vi "reward_behavior_timeout_phase1_2.vi"() -> ()   [LabVIEW 2019]
doc: "The myRIO Project template acquires acceleration data from the onboard accelerometer and displays the changes of acceleration values in a waveform chart."
uses:
  <vilib>/Analysis/Matrix/Datatypes/RealMatrix.ctl
  <vilib>/myRIO/Common/Instrument Driver Framework/myRIO v1.0/Encoder/typedefs/Encoder Signal Mode.ctl
  <vilib>/myRIO/Instrument Drivers/Onboard IO/Encoder/typedefs/Encoder Reference.ctl
  <vilib>/myRIO/Common/Instrument Driver Framework/Utilities/typedefs/myRIO Generic Hardware Reference.ctl
  <vilib>/myRIO/Common/Instrument Driver Framework/Utilities/typedefs/Hardware Version Enum.ctl
  <vilib>/myRIO/Common/Instrument Driver Framework/Utilities/typedefs/myRIO v1.0 Reference.ctl
  <vilib>/myRIO/Common/Instrument Driver Framework/Utilities/typedefs/Generic FPGA Reference.ctl
  <vilib>/myRIO/Common/Instrument Driver Framework/myRIO v1.0/Encoder/typedefs/Encoder Channels Enum.ctl
  <vilib>/myRIO/Common/Instrument Driver Framework/myRIO v1.0/Encoder/typedefs/Encoder Configuration v1.0.ctl
  <vilib>/userdefined/High Color/nirio_resource_hc.ctl
  <vilib>/myRIO/Instrument Drivers/Onboard IO/DIO/typedefs/DIO Reference.ctl
  <vilib>/myRIO/Common/Instrument Driver Framework/myRIO v1.0/DIO/typedefs/DIO Channels List.ctl
  <vilib>/myRIO/Common/Instrument Driver Framework/myRIO v1.0/DIO/typedefs/DIO Channels Enum.ctl
  <vilib>/myRIO/Common/Instrument Driver Framework/Utilities/vis/Is FPGA Ref Available.vi
  <vilib>/myRIO/Common/Instrument Driver Framework/myRIO v1.0/Encoder/vis/myRIO v1.1 Open Encoder.vi
  <vilib>/myRIO/Instrument Drivers/Onboard IO/Encoder/vis/Read.vi
  <vilib>/myRIO/Common/Instrument Driver Framework/myRIO v1.0/DIO/vis/myRIO v1.1 Open DIO.vi
  <vilib>/myRIO/Instrument Drivers/Onboard IO/DIO/vis/Write.vi
  <vilib>/myRIO/Instrument Drivers/Onboard IO/DIO/vis/Read.vi
  <vilib>/myRIO/Common/Instrument Driver Framework/Utilities/vis/Validate Channels.vi
  <vilib>/myRIO/Common/Instrument Driver Framework/myRIO v1.0/Encoder/vis/myRIO v1.0 Reserve Encoder.vi
  <vilib>/myRIO/Common/Instrument Driver Framework/myRIO v1.0/DIO/vis/myRIO v1.0 Reserve DIO.vi
  <vilib>/myRIO/Common/Instrument Driver Framework/myRIO v1.0/Encoder/vis/myRIO v1.0 Build MUX Configuration Encoder.vi
  <vilib>/myRIO/Common/Instrument Driver Framework/myRIO v1.0/Resource Manager/vis/myRIO v1.0 Reserve Channel List.vi
  <vilib>/myRIO/Common/Instrument Driver Framework/myRIO v1.0/DIO/vis/myRIO v1.0 Build MUX Configuration DIO.vi
  <vilib>/myRIO/Common/Instrument Driver Framework/myRIO v1.0/Resource Manager/vis/myRIO v1.0 Create Configuration List.vi
  <vilib>/myRIO/Common/Instrument Driver Framework/myRIO v1.0/Resource Manager/vis/myRIO v1.0 Reserve Channel.vi
  <vilib>/myRIO/Common/Instrument Driver Framework/myRIO v1.0/Resource Manager/vis/myRIO v1.0 Unreserve Channel.vi
  <vilib>/myRIO/Common/Instrument Driver Framework/myRIO v1.0/Resource Manager/vis/myRIO v1.0 Build Mutex Name.vi
  <vilib>/Utility/VariantDataType/GetNumericInfo.vi
  <vilib>/Utility/error.llb/Error Cluster From Error Code.vi
  <vilib>/myRIO/Common/Instrument Driver Framework/myRIO v1.0/myRIO v1.1 Open.vi
  <vilib>/myRIO/Common/Instrument Driver Framework/Utilities/vis/IO Manager.vi
  <vilib>/myRIO/Common/Instrument Driver Framework/Utilities/vis/Configuration Manager.vi
  <vilib>/myRIO/Common/Instrument Driver Framework/myRIO v1.0/Resource Manager/vis/myRIO v1.0 Configure IO.vi
  <vilib>/myRIO/Common/Instrument Driver Framework/myRIO v1.0/myRIO v1.0 Close.vi
  <vilib>/myRIO/Common/Instrument Driver Framework/myRIO v1.0/Encoder/vis/myRIO v1.0 Configure Encoder.vi
  <vilib>/myRIO/Common/Instrument Driver Framework/myRIO v1.0/Encoder/vis/myRIO v1.0 Read Encoder.vi
  <vilib>/myRIO/Common/Instrument Driver Framework/myRIO v1.0/DIO/vis/myRIO v1.0 Read DIO.vi
  <vilib>/myRIO/Common/Instrument Driver Framework/myRIO v1.0/DIO/vis/myRIO v1.0 Write DIO.vi
  <vilib>/myRIO/Express VI/Onboard IO/Encoder/Encoder Express VI.xnode
  <vilib>/myRIO/Instrument Drivers/Onboard IO/Encoder/vis/myRIO Encoder Open.xnode
  <vilib>/myRIO/Express VI/Onboard IO/DI/DI Express VI.xnode
  <vilib>/myRIO/Instrument Drivers/Onboard IO/DIO/vis/myRIO DIO Open.xnode
  <vilib>/myRIO/Express VI/Onboard IO/DO/DO Express VI.xnode
  <vilib>/myRIO/Instrument Drivers/Onboard IO/Encoder/Encoder.lvlib
  <vilib>/myRIO/Instrument Drivers/Onboard IO/DIO/DIO.lvlib
  <vilib>/Analysis/Matrix/NI_Matrix.lvlib
panel:
  out "Timings":dbl[](array[numeric])
  out "ISI":dbl
  out "ISI start time":dbl
  out "Time_out":bool=TRUE
  out "Time since lick":dbl
  out "Time of last lick":dbl
  out "Rewarded trials":dbl[](array[numeric])
  out "Rewards":u16
  out "Active Trial":bool
  out "Array temp2":T1
  out "Stimuli Loaded":bool
  out "Stim_ID":dbl[](array[numeric])
  out "Reward_mat":dbl[](array[numeric])
  out "Reward":bool=TRUE
  out "Frame clock":i32
  out "Licks":u32
  out "Lick":bool
  out "Time":dbl
  out "Stop":bool
  in  "Frames to collect":u32
  out "Overflow?":bool
  out "Counter Value":i32
  out "Velocity":dbl
  out "Velocity Plot":dbl[](graph)
  out "Velocity array":dbl[](array[numeric])
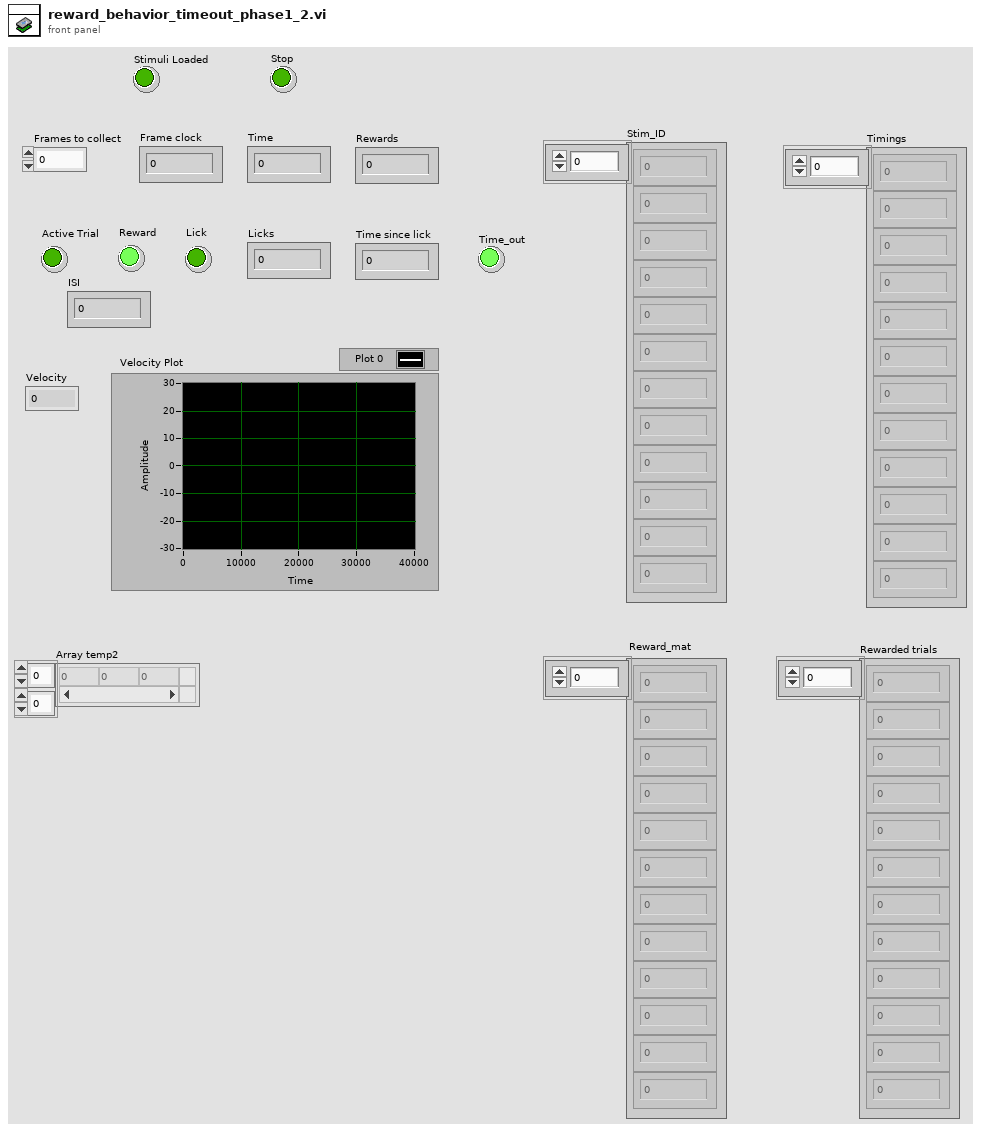
[diagram p1: front panel]
types:
  T1 = typedef "NI_Matrix.lvlib/RealMatrix.ctl" = dbl[][]
  T2 = typedef "Encoder.lvlib/Encoder Reference.ctl" = cluster{"myRIO Reference":T3, "Encoder Channels Enum":T7}
  T3 = typedef "myRIO Generic Hardware Reference.ctl" = cluster{"myRIO Model":T4, "myRIO Hardware Reference":T5}
  T4 = typedef "Hardware Version Enum.ctl" = enum16{"Unknown", "myRIO-1900", "myRIO-1950", "roboRIO", "NI ELVIS RIO CM", "ELVIS III"}
  T5 = typedef "myRIO v1.0 Reference.ctl" = cluster{"Generic FPGA Reference":T6, "Allow multiple opens":bool}
  T6 = typedef "Generic FPGA Reference.ctl" = refnum<k20>
  T7 = typedef "Encoder Channels Enum.ctl" = enum16{"Not Connected", "C/ENC0", "C/ENC1", "A/ENC", "A/ENC0", "A/ENC1", "A/ENC2", "A/ENC3", "A/ENC4", "A/ENC5", "A/ENC6", "A/ENC7", "A/ENC8", "A/ENC9", "B/ENC", "B/ENC0", "B/ENC1", "B/ENC2", "B/ENC3", "B/ENC4", "B/ENC5", "B/ENC6", "B/ENC7", "B/ENC8", "B/ENC9", "DIO/ENC0", "DIO/ENC1", "DIO/ENC2", "DIO/ENC3", "DIO/ENC4"}
  T8 = typedef "Encoder Signal Mode.ctl" = enum16{"Quadrature phase signal", "Step and direction signal"}
  T9 = typedef "nirio_resource_hc.ctl" = tag
  T10 = typedef "DIO.lvlib/DIO Reference.ctl" = cluster{"myRIO Reference":T3, "DIO Channels List":T11}
  T11 = typedef "DIO Channels List.ctl" = T12[]
  T12 = typedef "DIO Channels Enum.ctl" = enum16{"Not Connected", "C/DIO0", "C/DIO1", "C/DIO2", "C/DIO3", "C/DIO4", "C/DIO5", "C/DIO6", "C/DIO7", "A/DIO0", "A/DIO1", "A/DIO2", "A/DIO3", "A/DIO4", "A/DIO5", "A/DIO6", "A/DIO7", "A/DIO8", "A/DIO9", "A/DIO10", "A/DIO11", "A/DIO12", "A/DIO13", "A/DIO14", "A/DIO15", "A/DIO16", "A/DIO17", "A/DIO18", "A/DIO19", "B/DIO0", "B/DIO1", "B/DIO2", "B/DIO3", "B/DIO4", "B/DIO5", "B/DIO6", "B/DIO7", "B/DIO8", "B/DIO9", "B/DIO10", "B/DIO11", "B/DIO12", "B/DIO13", "B/DIO14", "B/DIO15", "B/DIO16", "B/DIO17", "B/DIO18", "B/DIO19", "LED0", "LED1", "LED2", "LED3", "Button0", "DIO/DIO0", "DIO/DIO1", "DIO/DIO2", "DIO/DIO3", "DIO/DIO4", "DIO/DIO5", "DIO/DIO6", "DIO/DIO7", "DIO/DIO8", "DIO/DIO9", "SPI/CS0", "SPI/CS1", "SPI/CS2", "SPI/CS3", "LED RADIO (Green)", "LED RADIO (Red)", "LED COMM (Green)", "LED COMM (Red)", "LED MODE (Green)", "LED MODE (Red)"}
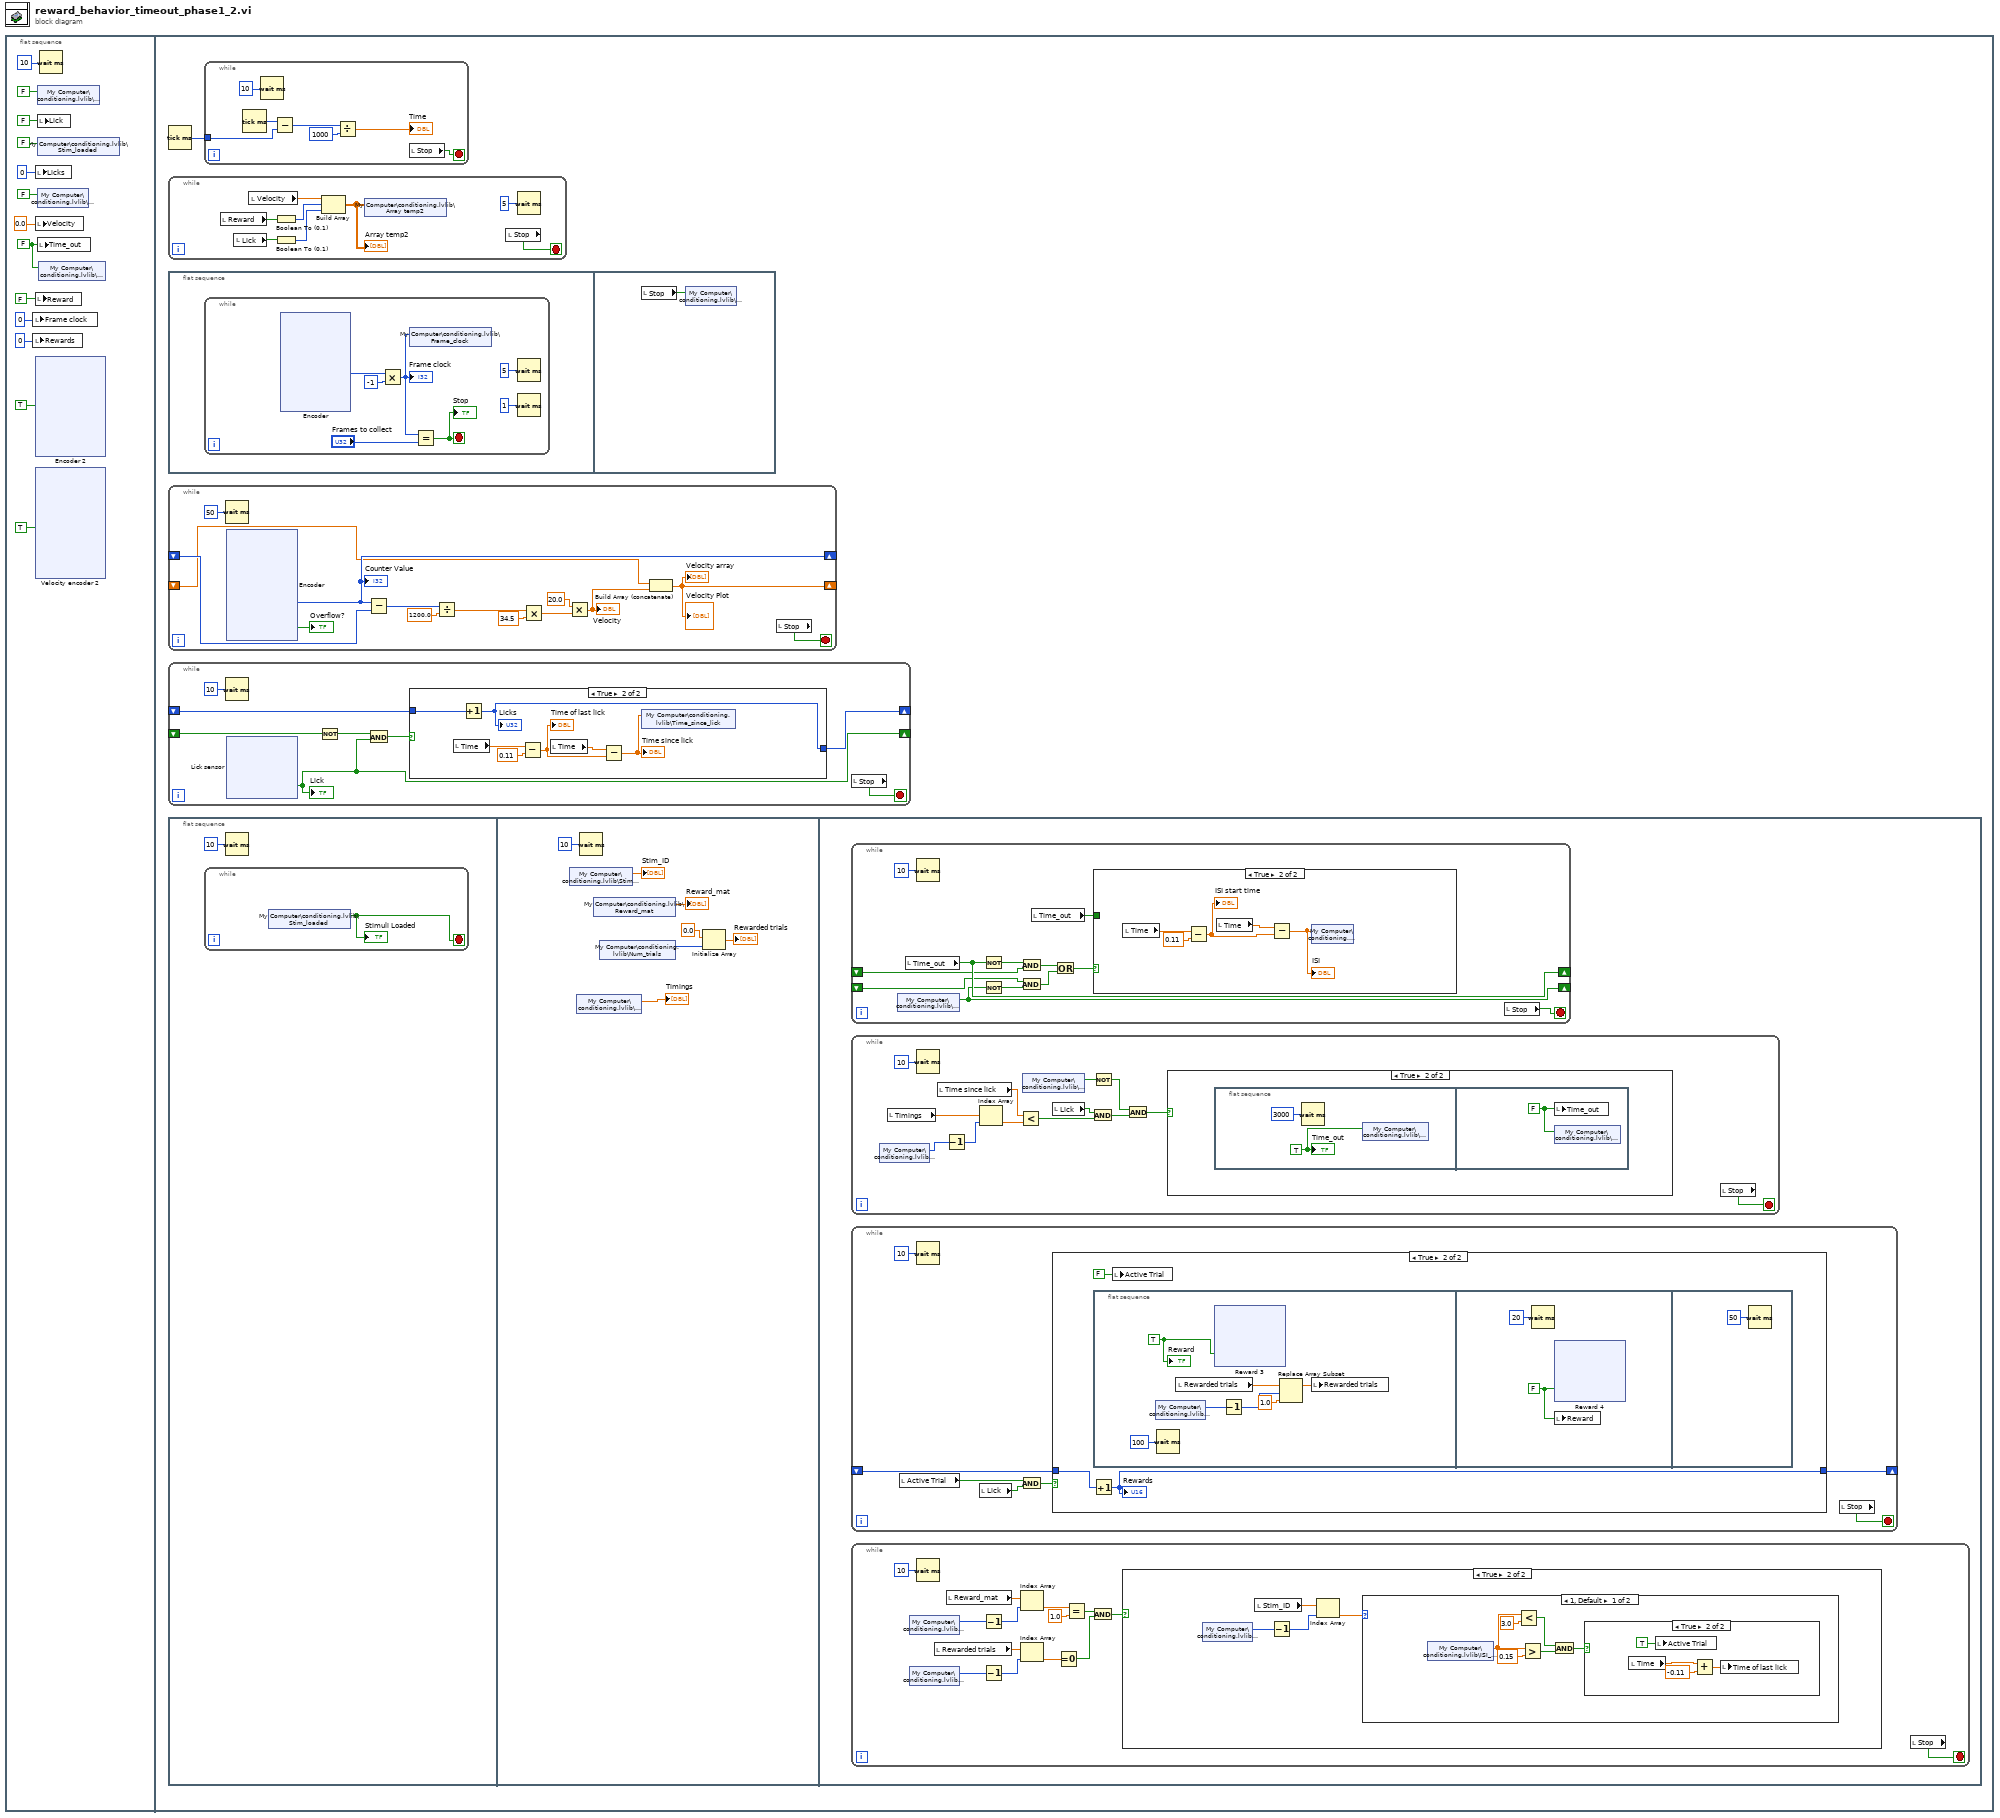
[diagram p0: block diagram]
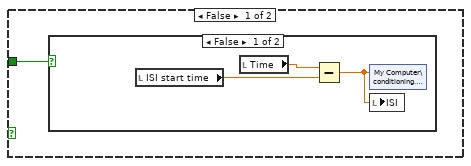
[diagram p3: hidden frame]
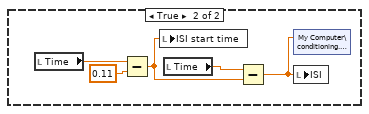
[diagram p4: hidden frame]
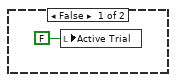
[diagram p5: hidden frame]
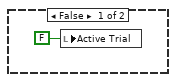
[diagram p6: hidden frame]
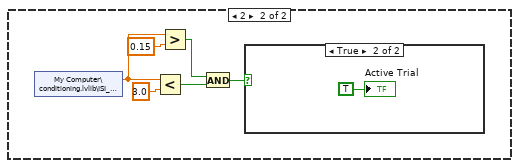
[diagram p7: hidden frame]
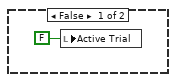
[diagram p8: hidden frame]
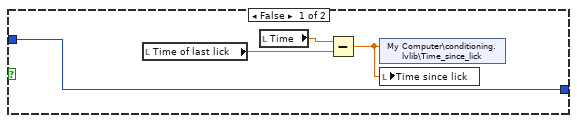
[diagram p10: hidden frame]
diagram:
  n1 = flat-sequence {
    frame #0 {
      w1 = FALSE ("Time_out")
      n2 = local write "Frame clock"(u32 0 ("Frames")) -> ()
      n3 = local write "Rewards"(u16 0 ("Rewards")) -> ()
      n4 = local write "Licks"(u32 0 ("Licks")) -> ()
      n5 = local write "Velocity"(0.0 ("Velocity")) -> ()
      n6 = local write "Reward"(FALSE ("Give reward")) -> ()
      n7 = xnode "Encoder 2"("Reset Counter"=TRUE) -> ()  [unwired: 1 in, 4 out]
      n8 = xnode "Velocity encoder 2"("Reset Counter"=TRUE) -> ()  [unwired: 1 in, 4 out]
      n9 = shared-variable "My Computer\\conditioning.lvlib\\Display"(FALSE ("Display")) -> ()  [unwired: 1 in, 1 out]
      n10 = local write "Lick"(FALSE ("Lick")) -> ()
      n11 = shared-variable "My Computer\\conditioning.lvlib\\Stim_loaded"(FALSE ("Stim_loaded")) -> ()  [unwired: 1 in, 1 out]
      n12 = shared-variable "My Computer\\conditioning.lvlib\\Stop"(FALSE ("Stop")) -> ()  [unwired: 1 in, 1 out]
      n13 = local write "Time_out"(w1) -> ()
      n14 = shared-variable "My Computer\\conditioning.lvlib\\Timeout"(w1) -> ()  [unwired: 1 in, 1 out]
      n15 = Wait (ms)(milliseconds to wait=u32 10) -> ()  [unwired: 1 out]
    }
    frame #1 {
      n16 = Tick Count (ms)() -> (millisecond timer value=w106:u32)
      n17 = while {
        stop <- w108 stop-if-true
        n18 = local read "Reward"() -> (w113:bool)
        n19 = local read "Lick"() -> (w114:bool)
        n20 = local read "Velocity"() -> (w112:dbl)
        n21 = Boolean To (0,1)(Boolean=w113) -> (0, 1=w111:i16)
        n22 = Boolean To (0,1)(Boolean=w114) -> (0, 1=w110:i16)
        n23 = Build Array(w112, w111, w110) -> (w107:T1)
        "Array temp2" <- w107
        n24 = shared-variable "My Computer\\conditioning.lvlib\\Array temp2"(w107) -> ()  [unwired: 1 in, 1 out]
        n25 = local read "Stop"() -> (w108:bool)
        n26 = Wait (ms)(milliseconds to wait=u32 5) -> ()  [unwired: 1 out]
      }
      n27 = flat-sequence {
        frame #0 {
          n28 = while {
            stop <- w296 stop-if-true
            n29 = xnode "Encoder"() -> ("Counter Value"=w300:i32)  [unwired: 2 in, 3 out]
            n30 = Multiply(x=w300, y=-1) -> (x*y=w295:i32)
            "Frame clock" <- w295
            n31 = shared-variable "My Computer\\conditioning.lvlib\\Frame_clock"(w295) -> ()  [unwired: 1 in, 1 out]
            n32 = Equal?(x=w295, y="Frames to collect") -> (x = y?=w296:bool)
            "Stop" <- w296
            n33 = Wait (ms)(milliseconds to wait=u32 5) -> ()  [unwired: 1 out]
            n34 = Wait (ms)(milliseconds to wait=u32 1) -> ()  [unwired: 1 out]
          }
        }
        frame #1 {
          n35 = local read "Stop"() -> (w348:bool)
          n36 = shared-variable "My Computer\\conditioning.lvlib\\Stop"(w348) -> ()  [unwired: 1 in, 1 out]
        }
      }
      n37 = while {
        shift-right: [w413] -> _
        shift-left: _ -> [w414]
        shift-right: [w405] -> _
        shift-left: _ -> [w404]
        stop <- w403 stop-if-true
        n38 = Wait (ms)(milliseconds to wait=u32 50) -> ()  [unwired: 1 out]
        n39 = xnode "Encoder"() -> ("Counter Value"=w413:i32, "Overflow?"=→"Overflow?":bool)  [unwired: 2 in, 2 out]
        "Counter Value" <- w413
        n40 = Subtract(x=w413, y=w414) -> (x-y=w406:i32)
        n41 = Divide(x=w406, y=1200.0 ("600")) -> (x/y=w411:dbl)
        n42 = Multiply(x=w411, y=34.5) -> (x*y=w409:dbl)
        n43 = Multiply(x=20.0, y=w409) -> (x*y=w407:dbl)
        "Velocity" <- w407
        n44 = Build Array (concatenate)(w404, w407) -> (w405:dbl[])
        "Velocity Plot" <- w405
        "Velocity array" <- w405
        n45 = local read "Stop"() -> (w403:bool)
      }
      n46 = while {
        shift-right: [w355] -> _
        shift-left: _ -> [w354]
        shift-right: [w349] -> _
        shift-left: _ -> [w352]
        stop <- w353 stop-if-true
        n47 = Wait (ms)(milliseconds to wait=u32 10) -> ()  [unwired: 1 out]
        n48 = xnode "Lick sensor"() -> ("C/DIO1 (DIO1)"=w349:bool)  [unwired: 1 in, 1 out]
        "Lick" <- w349
        n49 = Not(x=w352) -> (.not. x?=w351:bool)
        n50 = And(x=w351, y=w349) -> (x .and. y?=w350:bool)
        n51 = case shown="True" w350 {
          tunnel: [w360 w367] -> w355
          tunnel: w354 -> [w360 w366]
          frame False {
            n52 = local read "Time of last lick"() -> (w358:dbl)
            n53 = local read "Time"() -> (w359:dbl)
            n54 = Subtract(x=w359, y=w358) -> (x-y=w357:dbl)
            n55 = shared-variable "My Computer\\conditioning.lvlib\\Time_since_lick"(w357) -> ()  [unwired: 1 in, 1 out]
            n56 = local write "Time since lick"(w357) -> ()
          }
          frame True {
            n57 = local read "Time"() -> (w363:dbl)
            n58 = Increment(x=w366) -> (x+1=w367:u32)
            "Licks" <- w367
            n59 = Subtract(x=w363, y=0.11) -> (x-y=w361:dbl)
            "Time of last lick" <- w361
            n60 = local read "Time"() -> (w365:dbl)
            n61 = Subtract(x=w365, y=w361) -> (x-y=w364:dbl)
            "Time since lick" <- w364
            n62 = shared-variable "My Computer\\conditioning.lvlib\\Time_since_lick"(w364) -> ()  [unwired: 1 in, 1 out]
          }
        }
        n63 = local read "Stop"() -> (w353:bool)
      }
      n64 = flat-sequence {
        frame #0 {
          n65 = while {
            stop <- w116 stop-if-true
            n66 = shared-variable "My Computer\\conditioning.lvlib\\Stim_loaded"() -> (w116:bool)  [unwired: 1 in, 1 out]
            "Stimuli Loaded" <- w116
          }
          n67 = Wait (ms)(milliseconds to wait=u32 10) -> ()  [unwired: 1 out]
        }
        frame #1 {
          n68 = shared-variable "My Computer\\conditioning.lvlib\\Stim_ID"() -> (→"Stim_ID":dbl[])  [unwired: 1 in, 1 out]
          n69 = shared-variable "My Computer\\conditioning.lvlib\\Timings"() -> (→"Timings":dbl[])  [unwired: 1 in, 1 out]
          n70 = Wait (ms)(milliseconds to wait=u32 10) -> ()  [unwired: 1 out]
          n71 = shared-variable "My Computer\\conditioning.lvlib\\Reward_mat"() -> (→"Reward_mat":dbl[])  [unwired: 1 in, 1 out]
          n72 = shared-variable "My Computer\\conditioning.lvlib\\Num_trials"() -> (w120:u32)  [unwired: 1 in, 1 out]
          n73 = Initialize Array(0.0 ("element"), w120) -> (→"Rewarded trials":dbl[])
        }
        frame #2 {
          n74 = while {
            shift-right: [w150] -> _
            shift-left: _ -> [w148]
            shift-right: [w146] -> _
            shift-left: _ -> [w145]
            stop <- w151 stop-if-true
            n75 = shared-variable "My Computer\\conditioning.lvlib\\Display"() -> (w146:bool)  [unwired: 1 in, 1 out]
            n76 = local read "Time_out"() -> (w150:bool)
            n77 = Wait (ms)(milliseconds to wait=u32 10) -> ()  [unwired: 1 out]
            n78 = Not(x=w150) -> (.not. x?=w149:bool)
            n79 = Not(x=w146) -> (.not. x?=w144:bool)
            n80 = And(x=w149, y=w148) -> (x .and. y?=w143:bool)
            n81 = And(x=w145, y=w144) -> (x .and. y?=w142:bool)
            n82 = local read "Time_out"() -> (w147:bool)
            n83 = Or(x=w143, y=w142) -> (x .or. y?=w141:bool)
            n84 = case shown="True" w141 {
              tunnel: w147 -> [w152 _]
              frame False {
                n85 = case shown="False" w152 {
                  frame False {
                    n86 = local read "ISI start time"() -> (w155:dbl)
                    n87 = local read "Time"() -> (w154:dbl)
                    n88 = Subtract(x=w154, y=w155) -> (x-y=w153:dbl)
                    n89 = shared-variable "My Computer\\conditioning.lvlib\\ISI"(w153) -> ()  [unwired: 1 in, 1 out]
                    n90 = local write "ISI"(w153) -> ()
                  }
                  frame True {
                    n91 = local read "Time"() -> (w160:dbl)
                    n92 = Subtract(x=w160, y=0.11) -> (x-y=w157:dbl)
                    n93 = local write "ISI start time"(w157) -> ()
                    n94 = local read "Time"() -> (w158:dbl)
                    n95 = Subtract(x=w158, y=w157) -> (x-y=w156:dbl)
                    n96 = shared-variable "My Computer\\conditioning.lvlib\\ISI"(w156) -> ()  [unwired: 1 in, 1 out]
                    n97 = local write "ISI"(w156) -> ()
                  }
                }
              }
              frame True {
                n98 = local read "Time"() -> (w165:dbl)
                n99 = Subtract(x=w165, y=0.11) -> (x-y=w162:dbl)
                "ISI start time" <- w162
                n100 = local read "Time"() -> (w163:dbl)
                n101 = Subtract(x=w163, y=w162) -> (x-y=w161:dbl)
                "ISI" <- w161
                n102 = shared-variable "My Computer\\conditioning.lvlib\\ISI"(w161) -> ()  [unwired: 1 in, 1 out]
              }
            }
            n103 = local read "Stop"() -> (w151:bool)
          }
          n104 = while {
            stop <- w136 stop-if-true
            n105 = shared-variable "My Computer\\conditioning.lvlib\\Trial"() -> (w125:u32)  [unwired: 1 in, 1 out]
            n106 = local read "Timings"() -> (w127:dbl[])
            n107 = Wait (ms)(milliseconds to wait=u32 10) -> ()  [unwired: 1 out]
            n108 = local read "Time since lick"() -> (w135:dbl)
            n109 = Decrement(x=w125) -> (x-1=w124:u32)
            n110 = Index Array(array=w127, index=w124) -> (element=w126:dbl)
            n111 = Less?(x=w135, y=w126) -> (x < y?=w134:bool)
            n112 = shared-variable "My Computer\\conditioning.lvlib\\Display"() -> (w131:bool)  [unwired: 1 in, 1 out]
            n113 = local read "Lick"() -> (w133:bool)
            n114 = Not(x=w131) -> (.not. x?=w130:bool)
            n115 = And(x=w133, y=w134) -> (x .and. y?=w129:bool)
            n116 = And(x=w130, y=w129) -> (x .and. y?=w128:bool)
            n117 = case shown="True" w128 {
              frame False {
              }
              frame True {
                n118 = flat-sequence {
                  frame #0 {
                    w138 = TRUE
                    n119 = Wait (ms)(milliseconds to wait=u32 3000) -> ()  [unwired: 1 out]
                    n120 = shared-variable "My Computer\\conditioning.lvlib\\Timeout"(w138) -> ()  [unwired: 1 in, 1 out]
                    "Time_out" <- w138
                  }
                  frame #1 {
                    w139 = FALSE ("Timeout")
                    n121 = local write "Time_out"(w139) -> ()
                    n122 = shared-variable "My Computer\\conditioning.lvlib\\Timeout"(w139) -> ()  [unwired: 1 in, 1 out]
                  }
                }
              }
            }
            n123 = local read "Stop"() -> (w136:bool)
          }
          n124 = while {
            shift-right: [w207] -> _
            shift-left: _ -> [w206]
            stop <- w210 stop-if-true
            n125 = local read "Active Trial"() -> (w204:bool)
            n126 = Wait (ms)(milliseconds to wait=u32 10) -> ()  [unwired: 1 out]
            n127 = local read "Lick"() -> (w205:bool)
            n128 = And(x=w204, y=w205) -> (x .and. y?=w208:bool)
            n129 = case shown="True" w208 {
              tunnel: [w211 w214] -> w207
              tunnel: w206 -> [w211 w213]
              frame False {
              }
              frame True {
                n130 = Increment(x=w213) -> (x+1=w214:u16)
                "Rewards" <- w214
                n131 = flat-sequence {
                  frame #0 {
                    w220 = TRUE ("C/DIO0 (DIO0)")
                    n132 = shared-variable "My Computer\\conditioning.lvlib\\Trial"() -> (w219:u32)  [unwired: 1 in, 1 out]
                    n133 = Wait (ms)(milliseconds to wait=u32 100) -> ()  [unwired: 1 out]
                    n134 = local read "Rewarded trials"() -> (w217:dbl[])
                    n135 = xnode "Reward 3"("C/DIO0 (DIO0)"=w220) -> ()  [unwired: 1 in, 1 out]
                    n136 = Decrement(x=w219) -> (x-1=w218:u32)
                    n137 = Replace Array Subset(array=w217, new element=1.0 ("new element/subarray"), index=w218) -> (w215:dbl[])
                    n138 = local write "Rewarded trials"(w215) -> ()
                    "Reward" <- w220
                  }
                  frame #1 {
                    w258 = FALSE ("C/DIO0 (DIO0)")
                    n139 = Wait (ms)(milliseconds to wait=u32 20) -> ()  [unwired: 1 out]
                    n140 = xnode "Reward 4"("C/DIO0 (DIO0)"=w258) -> ()  [unwired: 1 in, 1 out]
                    n141 = local write "Reward"(w258) -> ()
                  }
                  frame #2 {
                    n142 = Wait (ms)(milliseconds to wait=u32 50) -> ()  [unwired: 1 out]
                  }
                }
                n143 = local write "Active Trial"(FALSE ("Active Trial")) -> ()
              }
            }
            n144 = local read "Stop"() -> (w210:bool)
          }
          n145 = while {
            stop <- w179 stop-if-true
            n146 = shared-variable "My Computer\\conditioning.lvlib\\Trial"() -> (w175:u32)  [unwired: 1 in, 1 out]
            n147 = shared-variable "My Computer\\conditioning.lvlib\\Trial"() -> (w171:u32)  [unwired: 1 in, 1 out]
            n148 = Wait (ms)(milliseconds to wait=u32 10) -> ()  [unwired: 1 out]
            n149 = local read "Rewarded trials"() -> (w172:dbl[])
            n150 = local read "Reward_mat"() -> (w174:dbl[])
            n151 = Decrement(x=w175) -> (x-1=w176:u32)
            n152 = Decrement(x=w171) -> (x-1=w170:u32)
            n153 = Index Array(array=w174, index=w176) -> (element=w177:dbl)
            n154 = Index Array(array=w172, index=w170) -> (element=w169:dbl)
            n155 = Equal To 0?(x=w169) -> (x = 0?=w168:bool)
            n156 = Equal?(x=w177, y=1.0) -> (x = y?=w167:bool)
            n157 = And(x=w167, y=w168) -> (x .and. y?=w166:bool)
            n158 = case shown="True" w166 {
              frame False {
                n159 = local write "Active Trial"(FALSE ("Active_trial")) -> ()
              }
              frame True {
                n160 = shared-variable "My Computer\\conditioning.lvlib\\Trial"() -> (w182:u32)  [unwired: 1 in, 1 out]
                n161 = local read "Stim_ID"() -> (w184:dbl[])
                n162 = Decrement(x=w182) -> (x-1=w183:u32)
                n163 = Index Array(array=w184, index=w183) -> (element=w181:dbl)
                n164 = case shown="1, Default" w181 {
                  frame 1, Default {
                    n165 = shared-variable "My Computer\\conditioning.lvlib\\ISI_Time"() -> (w189:dbl)  [unwired: 1 in, 1 out]
                    n166 = Less?(x=w189, y=3.0) -> (x < y?=w187:bool)
                    n167 = Greater?(x=w189, y=0.15) -> (0:w186:bool)
                    n168 = And(x=w187, y=w186) -> (x .and. y?=w185:bool)
                    n169 = case shown="True" w185 {
                      frame False {
                        n170 = local write "Active Trial"(FALSE ("Active Trial")) -> ()
                      }
                      frame True {
                        n171 = local read "Time"() -> (w194:dbl)
                        n172 = local write "Active Trial"(TRUE ("Active Trial")) -> ()
                        n173 = Add(x=w194, y=-0.11) -> (x+y=w192:dbl)
                        n174 = local write "Time of last lick"(w192) -> ()
                      }
                    }
                  }
                  frame 2 {
                    n175 = shared-variable "My Computer\\conditioning.lvlib\\ISI_Time"() -> (w200:dbl)  [unwired: 1 in, 1 out]
                    n176 = Less?(x=w200, y=3.0) -> (x < y?=w197:bool)
                    n177 = Greater?(x=w200, y=0.15) -> (0:w198:bool)
                    n178 = And(x=w198, y=w197) -> (x .and. y?=w196:bool)
                    n179 = case shown="True" w196 {
                      frame False {
                        n180 = local write "Active Trial"(FALSE ("Active Trial")) -> ()
                      }
                      frame True {
                        "Active Trial" <- TRUE ("Active Trial")
                      }
                    }
                  }
                }
              }
            }
            n181 = local read "Stop"() -> (w179:bool)
          }
        }
      }
      n182 = while {
        tunnel: w106 -> [w468]
        stop <- w466 stop-if-true
        n183 = Tick Count (ms)() -> (millisecond timer value=w469:u32)
        n184 = Wait (ms)(milliseconds to wait=u32 10) -> ()  [unwired: 1 out]
        n185 = Subtract(x=w469, y=w468) -> (x-y=w465:u32)
        n186 = Divide(x=w465, y=u32 1000) -> (x/y=→"Time":dbl)
        n187 = local read "Stop"() -> (w466:bool)
      }
    }
  }
